vi "Base_eleve.vi"() -> ()   [LabVIEW 2018]
uses:
  <vilib>/Instr/_visa.llb/VISA Configure Serial Port (Instr).vi
panel:
  in  "créer fichier":bool
  in  "emplacement du fichier":path
  in  "nom du fichier":string
  in  "stop":bool
  in  "Pause/Go":bool
  out "Humidity Chart":dbl(graph)
  out "Pressure Chart":dbl(graph)
  out "Temperature Chart":dbl(graph)
  out "Humidity":dbl
  out "Pressure":dbl
  out "Temperature":dbl
  out "Chaîne":string
  in  "Nom de ressource VISA":refnum<visa-resource-name>
  # "1. Brancher la carte Arduino sur un port USB\n2. Choisir le port COM de la carte dans la liste déroulante \"Nom de ressource VISA\"\n3. Lancer le programme"
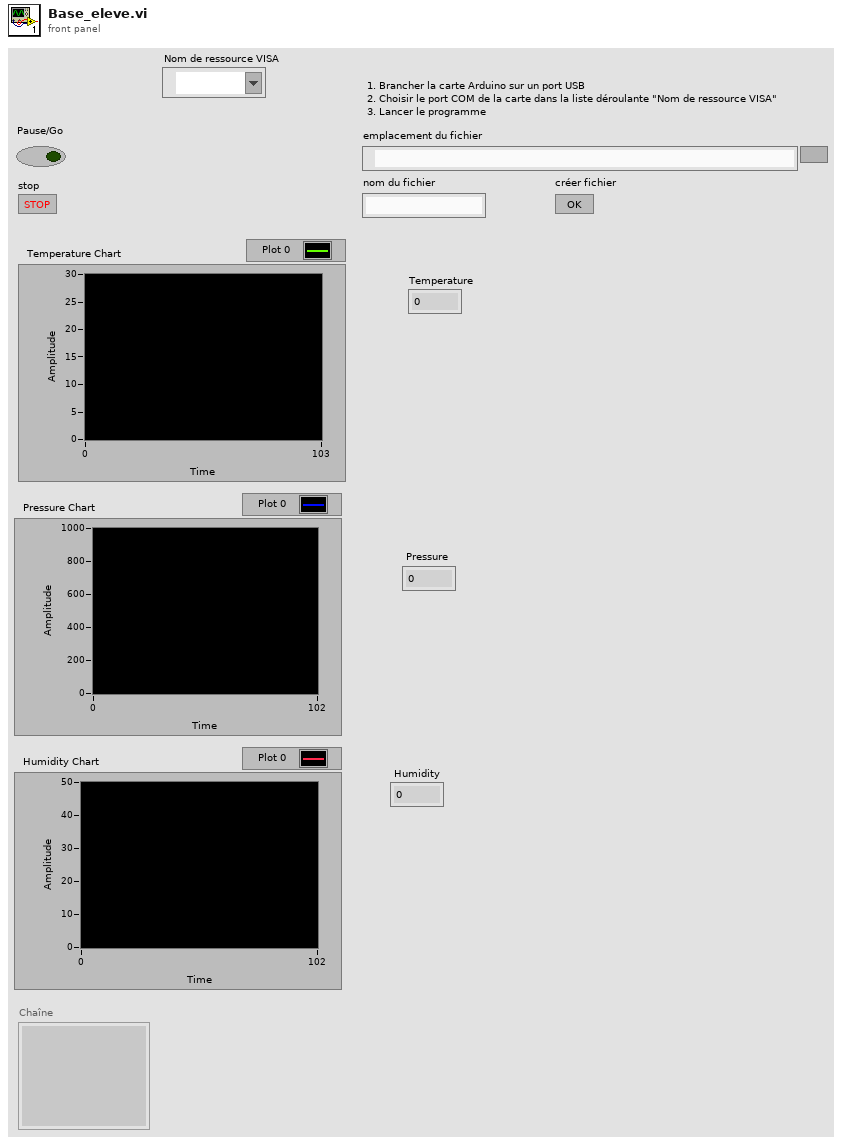
[diagram p1: front panel]
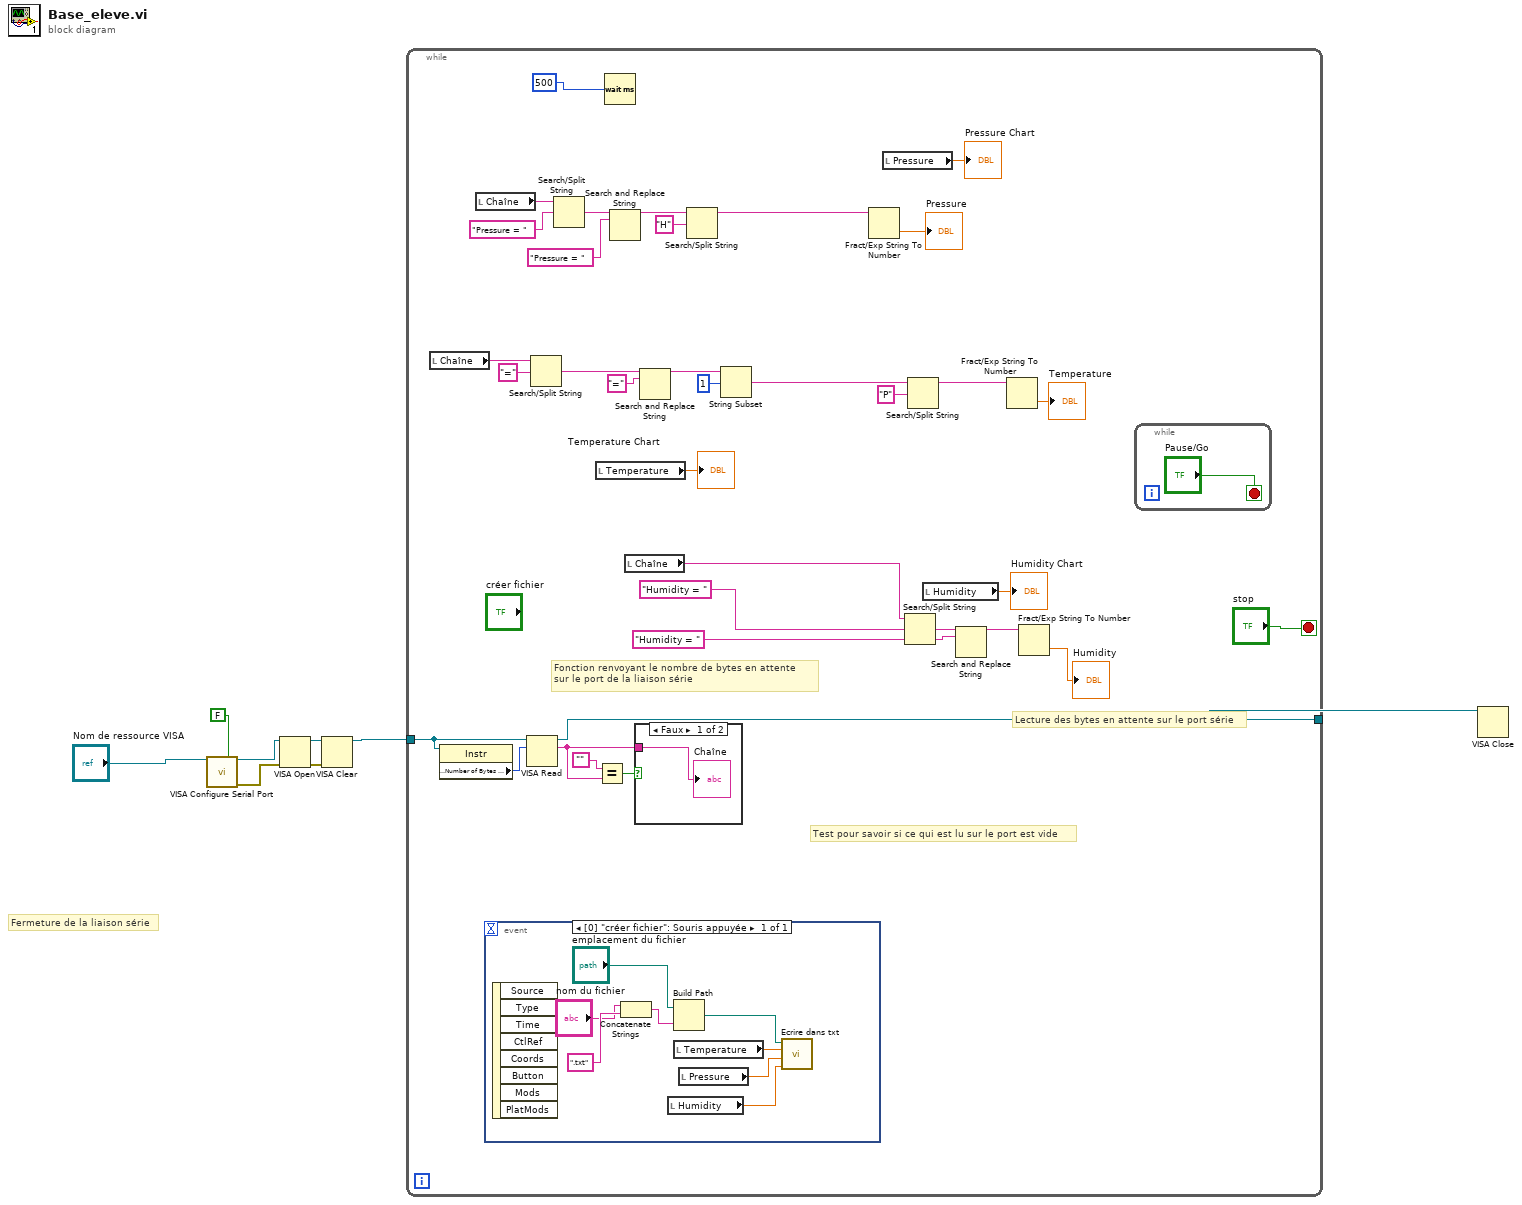
[diagram p0: block diagram]
diagram:
  # "Fermeture de la liaison série"
  n1 = call-poly "VISA Configure Serial Port"("VISA resource name"="Nom de ressource VISA", "Enable Termination\nChar (T)"=FALSE ("Enable Termination\nChar (T)")) -> ("VISA resource name out"=w4:refnum<visa-resource-name>, "error out"=w3:errorcluster)  [unwired: 12 in]
  n2 = VISA Open(error in (no error)=w3, VISA resource name=w4) -> (VISA resource name=w6:refnum<visa-resource-name>, error out=w2:errorcluster)  [unwired: 3 in]
  n3 = VISA Clear(VISA resource name=w6, error in (no error)=w2) -> (VISA resource name out=w5:refnum<visa-resource-name>)  [unwired: 1 out]
  n4 = while {
    tunnel: w5 -> [w43]
    tunnel: [w41] -> w1
    stop <- "stop" stop-if-true
    # "Lecture des bytes en attente sur le port série"
    # "Fonction renvoyant le nombre de bytes en attente\nsur le port de la liaison série"
    # "Test pour savoir si ce qui est lu sur le port est vide"
    n5 = local read "Chaîne"() -> (w30:string)
    n6 = property class="Instr"(reference=w43) -> ("Serial Settings:Number of Bytes at Serial Port"=w42:u32)  [unwired: 1 in, 2 out]
    n7 = local read "Chaîne"() -> (w19:string)
    n8 = event shown="[0] \"créer fichier\": Souris appuyée" {
      selector: _ -> [_]
      dyn-events: _ -> [_]
      timeout: _ -> [_]
      event "créer fichier": Mouse Down {
        n9 = event-data() -> ()  [unwired: 1 in, 8 out]
        n10 = Concatenate Strings("nom du fichier", ".txt") -> (w49:string)
        n11 = local read "Humidity"() -> (w44:dbl)
        n12 = Build Path(base path="emplacement du fichier", name or relative path=w49) -> (appended path=w47:path)
        n13 = local read "Temperature"() -> (w46:dbl)
        n14 = local read "Pressure"() -> (w45:dbl)
        n15 = call "Ecrire dans txt.vi"("Numeric 3"=w44, "Numeric 2"=w45, "Numeric"=w46, "Path"=w47) -> ()
      }
    }
    n16 = VISA Read(VISA resource name=w43, byte count=w42) -> (VISA resource name out=w41:refnum<visa-resource-name>, read buffer=w38:string)  [unwired: 1 in, 2 out]
    n17 = Search/Split String(string=w30, search string/char (-)="=") -> (match + rest of string=w29:string)  [unwired: 1 in, 2 out]
    n18 = Search/Split String(string=w19, search string/char (-)="Pressure = ") -> (match + rest of string=w18:string)  [unwired: 1 in, 2 out]
    n19 = local read "Temperature"() -> (→"Temperature Chart":dbl)
    n20 = Equal?(x="", y=w38) -> (x = y?=w39:bool)
    n21 = Wait (ms)(milliseconds to wait=500) -> ()  [unwired: 1 out]
    n22 = Search and Replace String(input string=w18, search string="Pressure = ") -> (result string=w17:string)  [unwired: 6 in, 3 out]
    n23 = local read "Chaîne"() -> (w36:string)
    n24 = case shown="Faux" w39 {
      tunnel: w38 -> [w53 _]
      frame False {
        "Chaîne" <- w53
      }
      frame True {
      }
    }
    n25 = Search and Replace String(input string=w29, search string="=") -> (result string=w28:string)  [unwired: 6 in, 3 out]
    n26 = Search/Split String(string=w17, search string/char (-)="H") -> (substring before match=w16:string)  [unwired: 1 in, 2 out]
    n27 = String Subset(string=w28, offset (0)=1) -> (substring=w27:string)  [unwired: 1 in]
    n28 = Fract/Exp String To Number(string=w16) -> (number=→"Pressure":dbl)  [unwired: 3 in, 1 out]
    n29 = local read "Pressure"() -> (→"Pressure Chart":dbl)
    n30 = Search/Split String(string=w36, search string/char (-)="Humidity = ") -> (match + rest of string=w37:string)  [unwired: 1 in, 2 out]
    n31 = Search/Split String(string=w27, search string/char (-)="P") -> (substring before match=w26:string)  [unwired: 1 in, 2 out]
    n32 = local read "Humidity"() -> (→"Humidity Chart":dbl)
    n33 = Search and Replace String(input string=w37, search string="Humidity = ") -> (result string=w35:string)  [unwired: 6 in, 3 out]
    n34 = Fract/Exp String To Number(string=w26) -> (number=→"Temperature":dbl)  [unwired: 3 in, 1 out]
    n35 = Fract/Exp String To Number(string=w35) -> (number=→"Humidity":dbl)  [unwired: 3 in, 1 out]
    n36 = while {
      stop <- "Pause/Go" stop-if-true
    }
  }
  n37 = VISA Close(VISA resource name=w1) -> ()  [unwired: 1 in, 1 out]
